vi "Fluke 28x Series Channel Summation.vi"() -> ()   [LabVIEW 2015]
doc: "This example shows how to configure and sum two channels together."
uses:
  <instrlib>/Fluke 28x Series/Fluke 28x Series.lvlib
panel:
  in  "Waveform Function (0: Sine)":u16(ring) items=["Sine", "Square", "Triangle", "Cosine", "DC", "Positive Ramp", "Negative Ramp", "Haversine", "Havercosine", "Sine (x)/x"]
  in  "Channel Ratio (0.5)":dbl=0.5
  in  "Channel Summation Source (0: External Sum)":u16(ring)=1 items=["External Sum", "Previous Channel"]
  in  "Channel (1)":u32(ring)=1 items=["1"=1, "2"=2, "3"=3, "4"=4]
  in  "Output Channel (1)":u32(ring)=1 items=["1"=1, "2"=2, "3"=3, "4"=4]
  in  "VISA resource name":refnum<visa-resource-name>
  # "(c) 2009-2014 National Instruments.  ALL RIGHTS RESERVED."
  # "Output Channel"
  # "Input/Sum Channel"
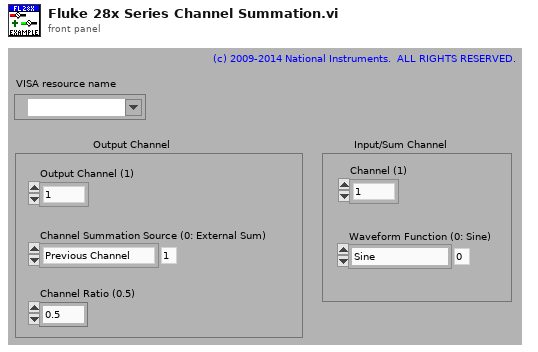
[diagram p1: front panel]
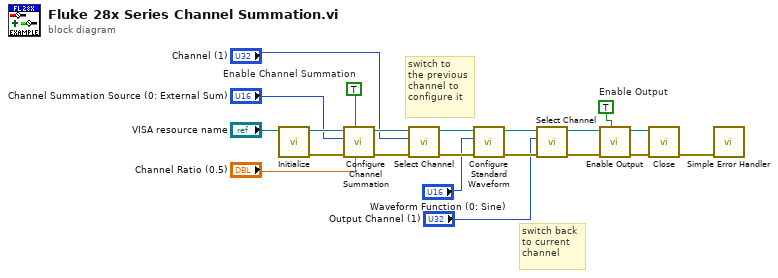
[diagram p0: block diagram]
diagram:
  w6 = TRUE  # Enable Channel Summation
  w5 = TRUE  # Enable Output
  # "switch back\nto current\nchannel"
  # "switch to \nthe previous\nchannel to\nconfigure it"
  n1 = call <instrlib>:"Initialize.vi"("VISA resource name"="VISA resource name") -> ("error out"=w19:errorcluster, "VISA resource name out"=w20:refnum<visa-resource-name>)  [unwired: 9 in]
  n2 = call <instrlib>:"Configure Channel Summation.vi"("Channel Ratio (0.5)"="Channel Ratio (0.5)", "Enable Channel Summation (T: Enable)"=w6, "error in (no error)"=w19, "Channel Summation Source (0: External Sum)"="Channel Summation Source (0: External Sum)", "VISA resource name"=w20) -> ("error out"=w16:errorcluster, "VISA resource name out"=w15:refnum<visa-resource-name>)  [unwired: 5 in]
  n3 = call <instrlib>:"Select Channel.vi"("error in (no error)"=w16, "Channel (1)"="Channel (1)", "VISA resource name"=w15) -> ("error out"=w17:errorcluster, "VISA resource name out"=w14:refnum<visa-resource-name>)  [unwired: 7 in]
  n4 = call <instrlib>:"Configure Standard Waveform.vi"("error in (no error)"=w17, "Waveform Function (0: Sine)"="Waveform Function (0: Sine)", "VISA resource name"=w14) -> ("error out"=w13:errorcluster, "VISA resource name out"=w12:refnum<visa-resource-name>)  [unwired: 7 in]
  n5 = call <instrlib>:"Select Channel.vi"("error in (no error)"=w13, "Channel (1)"="Output Channel (1)", "VISA resource name"=w12) -> ("error out"=w11:errorcluster, "VISA resource name out"=w10:refnum<visa-resource-name>)  [unwired: 7 in]
  n6 = call <instrlib>:"Enable Output.vi"("Enable Output (T: Enable)"=w5, "error in (no error)"=w11, "VISA resource name"=w10) -> ("error out"=w7:errorcluster, "VISA resource name out"=w8:refnum<visa-resource-name>)  [unwired: 7 in]
  n7 = call <instrlib>:"Close.vi"("error in (no error)"=w7, "VISA resource name"=w8) -> ("error out"=w18:errorcluster)  [unwired: 9 in]
  n8 = call <vilib>:"Simple Error Handler.vi"("error in (no error)"=w18) -> ()  [unwired: 4 in, 5 out]
